vi "Example Analog.vi"() -> ()   [LabVIEW 2022 SP3]
uses:
  Controls/SampleRateControlAin.ctl
  Controls/SampleRateControlOut.ctl
  Controls/AnalogChannel.ctl
  <vilib>/measure/NI_MAPro.lvlib
panel:
  in  "Stop Button":bool
  in  "DAC Samplerate":T1
  in  "formula for generated signal":string="sin(w*t)*sin(2*pi(1)*t)"
  in  "amplitude":dbl=1.0 format="%0.2p"
  in  "frequency":dbl=10.0 format="%0.2p"
  in  "Samples / channel ADC":i32=8192
  in  "Calibrate":bool=TRUE
  in  "ADC Samplerate (Hz)":T2
  out "CHANNEL 2 Plot":waveform(dbl)(graph)
  out "CHANNEL 1 Plot":waveform(dbl)(graph)
  in  "ADALM2000 URI:":string
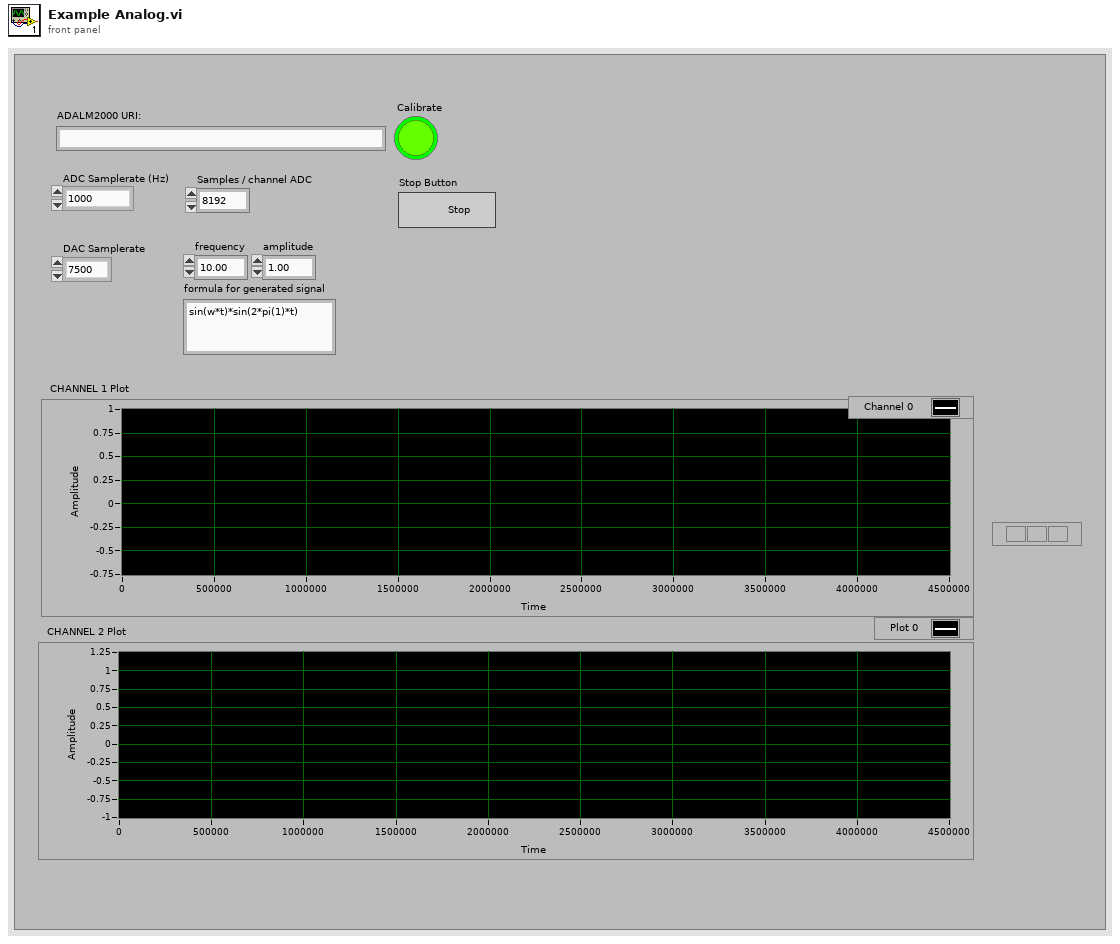
[diagram p1: front panel]
types:
  T1 = typedef "SampleRateControlOut.ctl" = enum16{"7500", "75000", "750000", "7500000", "75000000"}
  T2 = typedef "SampleRateControlAin.ctl" = enum16{"1000", "10000", "100000", "1000000", "10000000", "100000000"}
  T3 = typedef "AnalogChannel.ctl" = enum16{"ANALOG_CH_1", "ANALOG_CH_2"}
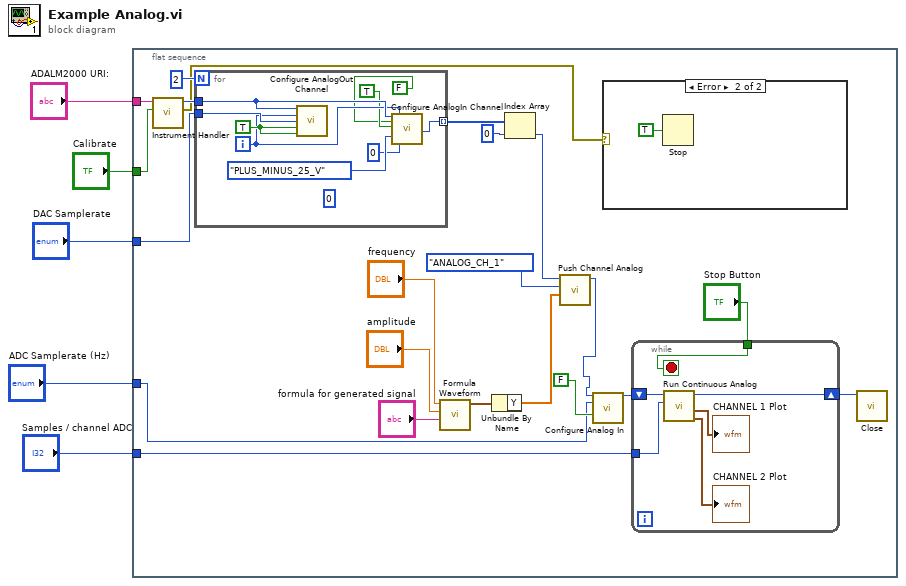
[diagram p0: block diagram]
diagram:
  n1 = flat-sequence {
    tunnel: "ADC Samplerate (Hz)" -> [w6]
    tunnel: "ADALM2000 URI:" -> [w23]
    tunnel: "Calibrate" -> [w22]
    tunnel: "Samples / channel ADC" -> [w14]
    tunnel: "DAC Samplerate" -> [w18]
    frame #0 {
      n2 = call "Instrument Handler.vi"("Calibrate"=w22, "ADALM2000 URI"=w23) -> ("error out"=w11:errorcluster, "ADALM2000 Handle"=w27:u64)  [unwired: 8 in]
      n3 = for {
        N: 2 -> [_]
        tunnel: w27 -> [w41]
        tunnel: [w40] -> w17 mode=indexing
        tunnel: w18 -> [w42]
        i -> [w37]
        (unwired) 0
        w43 = TRUE ("Enable")
        n4 = call "Configure AnalogOut Channel.vi"("ADALM2000 Handler"=w41, "Channel"=w37, "Samplerate"=w42, "Enable"=w43, "Cyclic"=w43) -> ()  [unwired: 10 in, 1 out]
        n5 = call "Configure AnalogIn Channel.vi"("ADALM2000 In"=w41, "Trigger enable"=FALSE, "Enable"=TRUE ("Trigger enable"), "Range"=enum16{"PLUS_MINUS_25_V", "PLUS_MINUS_2_5V"}."PLUS_MINUS_25_V", "Channel"=w37, "Vertical offset"=u64 0 ("Channel")) -> ("ADALM2000 Out"=w40:u64)  [unwired: 13 in]
      }
      n6 = call <vilib>:"Formula Waveform.vi"("formula"="formula for generated signal", "amplitude"="amplitude", "frequency"="frequency") -> ("signal out"=w10:waveform(dbl))  [unwired: 7 in, 1 out]
      n7 = Unbundle By Name(w10) -> ("Y"=w15:dbl[])
      n8 = Index Array(array=w17, index=0) -> (element=w16:u64)
      n9 = call "Push Channel Analog.vi"("ADALM2000 Handler"=w16, "Channel"=AnalogChannel."ANALOG_CH_1", "data"=w15) -> ("ADALM2000 Handler 2"=w9:u64)  [unwired: 7 in]
      n10 = call "Configure Analog In.vi"("ADALM2000 Handler"=w9, "Samplerate (Hz)"=w6, "Trigger enable"=FALSE) -> ("ADALM2000 Handler 2"=w8:u64)  [unwired: 12 in]
      n11 = case shown="Error" w11 {
        frame No Error {
        }
        frame Error {
          n12 = Stop(stop? (T)=TRUE) -> ()
        }
      }
      n13 = while {
        shift-right: [w34] -> w24
        shift-left: w8 -> [w33]
        tunnel: w14 -> [w30]
        tunnel: "Stop Button" -> [w29]
        stop <- w29 stop-if-true
        n14 = call "Run Continuous Analog.vi"("Samples / channel"=w30, "ADALM2000 Handler"=w33) -> ("Waveform 2"=→"CHANNEL 2 Plot":waveform(dbl), "Waveform"=→"CHANNEL 1 Plot":waveform(dbl), "ADALM2000 Handler 2"=w34:u64)  [unwired: 7 in]
      }
      n15 = call "Close.vi"("ADALM2000 Handler"=w24) -> ()  [unwired: 11 in]
    }
  }
